vi "FPGA_main_simplified_debug.vi"() -> ()   [LabVIEW 2024]
uses:
  <vilib>/Platform/TimedLoop/XDataNode/timing_clust.ctl
  <vilib>/Platform/TimedLoop/XDataNode/nitl_modes.ctl
  <vilib>/Platform/TimedLoop/XDataNode/wakeup.ctl
  <vilib>/LabVIEW Targets/FPGA/cRIO/shared/nicrio_ModuleControls/nicrio_cRIO-9775_ContinuousDataRates4ChansRing.ctl
  <vilib>/rvi/Emulation/niFpgaGetClockAttributes.vi
  <vilib>/rvi/Emulation/niFpgaSctlEmulationGetInTimedLoop.vi
  <vilib>/rvi/Emulation/niFpgaEmulationReportErrorSimple.vi
  <vilib>/rvi/Emulation/niFpgaProcessEmulError.vi
  <vilib>/rvi/eio/common/nirviEmuTemplateMethod_errors.vi
  <vilib>/rvi/Emulation/niFpgaCriticalErrorInLSC.vi
  <vilib>/rvi/eio/common/nirviEmuTemplatePropertySet_errors.vi
  <vilib>/eio/utilities/niEioResolveVilibRelativePath.vi
  <vilib>/rvi/interface/RandomDataEmulation/niFpgaRandomDataHandleErrors.vi
  <vilib>/eio/EIONode/EIONode.xnode
  <vilib>/eio/EIOMethodNode/EIOMethodNode.xnode
  <vilib>/eio/EIOPropertyNode/EIOPropertyNode.xnode
  <vilib>/platform/TimedLoop/XDataNode/XDataNode.xnode
  <vilib>/rvi/DataTransferAndStorage/Container/XNode/niFpgaContainer.xnode
  <vilib>/rvi/interface/RandomDataEmulation/nirviRandomDataFpgaReadWriteTemplate.vi
  <vilib>/Platform/TimedLoop/XDataNode/XDNodeRunTimeDep.lvlib
  <vilib>/rvi/eio/common/nirviEmuTemplatePropertyGet_errors.vi
  <vilib>/rvi/eio/common/nirviEmuTemplatePropertyGet_noerrors.vi
  <vilib>/rvi/eio/common/nirviEmuTemplatePropertySet_noerrors.vi
panel:
  out "Use Triggers":bool
  out "Tr FIFO Full":bool
  out "@Next R":u32
  out "Last Tr (R-F)":u32
  out "Current Data Cycle":u32
  out "Tr Finished":bool
  in  "Total Triggers":u32=10
  out "Current Trigger":u32
  out "FPGA routine\nrunning":bool
  in  "Pulse\nWidth":u32 caption="Pulse width(uSec)"
  in  "Pulse\nPeriod":u32 caption="Period(uSec)"
  in  "Stop Routine":bool
  in  "DIO3":bool
  in  "DIO2":bool
  in  "DIO1":bool
  in  "DIO0":bool
  out "Rebinned Counts":i32
  in  "Binning Time (ticks)":i32=1200000
  out "Counts":u8
  out "FPGA Error":errorcluster
  out "Finished":bool
  in  "Stop":bool
  out "Module Underflow":bool
  out "DMA FIFO Full":bool
  out "Actual Loop Period (ticks)":u32=40
  out "First Read":bool
  in  "Type Counter":enum16{"Falling Edge", "Rising Edge"}(ring)
  # "Photon counting. Single cycle time loop"
  # "User Control of digital output"
  # "Thresholding"
  # "Pulsing DIO 0 (Pulse width should be shorter than\n period)"
  # "Binning and streaming binned Total Count"
  # "Streaming Analog Input Data"
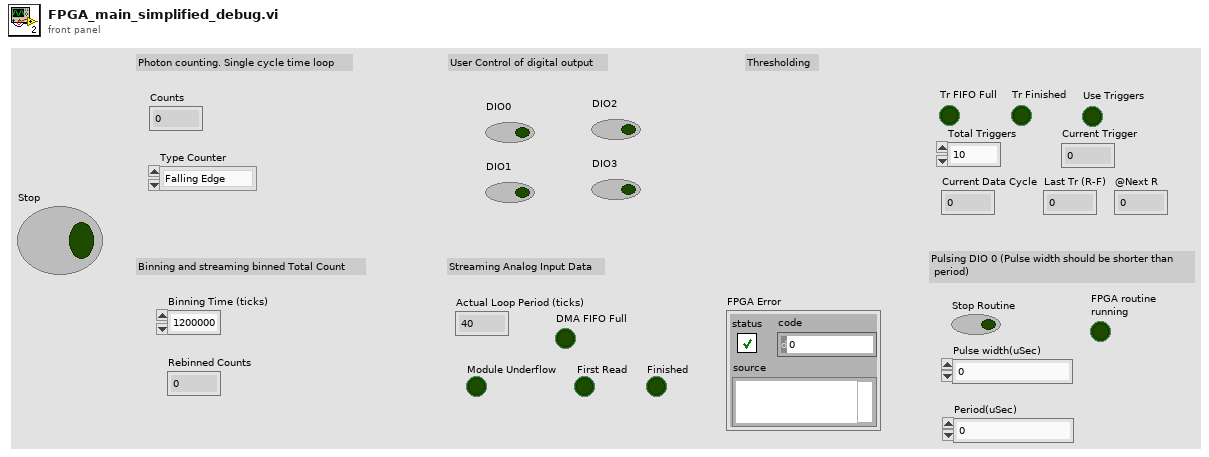
[diagram p1: front panel]
types:
  T1 = typedef "XDNodeRunTimeDep.lvlib/timing_clust.ctl" = cluster{"Expected End [f-1]":u64, "Actual End [f-1]":u64, "Finished Late? [f-1]":bool, "Expected End [i-1]":u64, "Actual End [i-1]":u64, "Finished Late? [i-1]":bool, "Expected Start [i]":u64, "Actual Start [i]":u64, "Expected Start [f]":u64, "Actual Start [f]":u64, "Source Name":string, "Structure Name":string, "Period":i64, "Deadline":i64, "Offset":i64, "Start":i64, "Priority":i32, "Timeout":i32, "Mode":T2, "Wakeup Reason":T3, "Error":errorcluster, "Source Type":string, "Secondary Source Type":string, "Global End Time":u64, "Global Start Time":u64, "Frame Duration":u64, "Iteration Duration":u64, "Assigned CPU":i32, "I/O Scan Engine Mode":u32}
  T2 = typedef "XDNodeRunTimeDep.lvlib/nitl_modes.ctl" = enum32{"No Change", "Process missed periods, maintain original phase", "Discard missed periods, maintain original phase", "Process missed periods, ignore original phase", "Discard missed periods, ignore original phase"}
  T3 = typedef "XDNodeRunTimeDep.lvlib/wakeup.ctl" = enum32{"Normal", "Aborted", "Asynchronous wakeup", "Timing source error", "Timed loop error", "Timeout"}
  T4 = typedef "nicrio_cRIO-9775_ContinuousDataRates4ChansRing.ctl" = u16
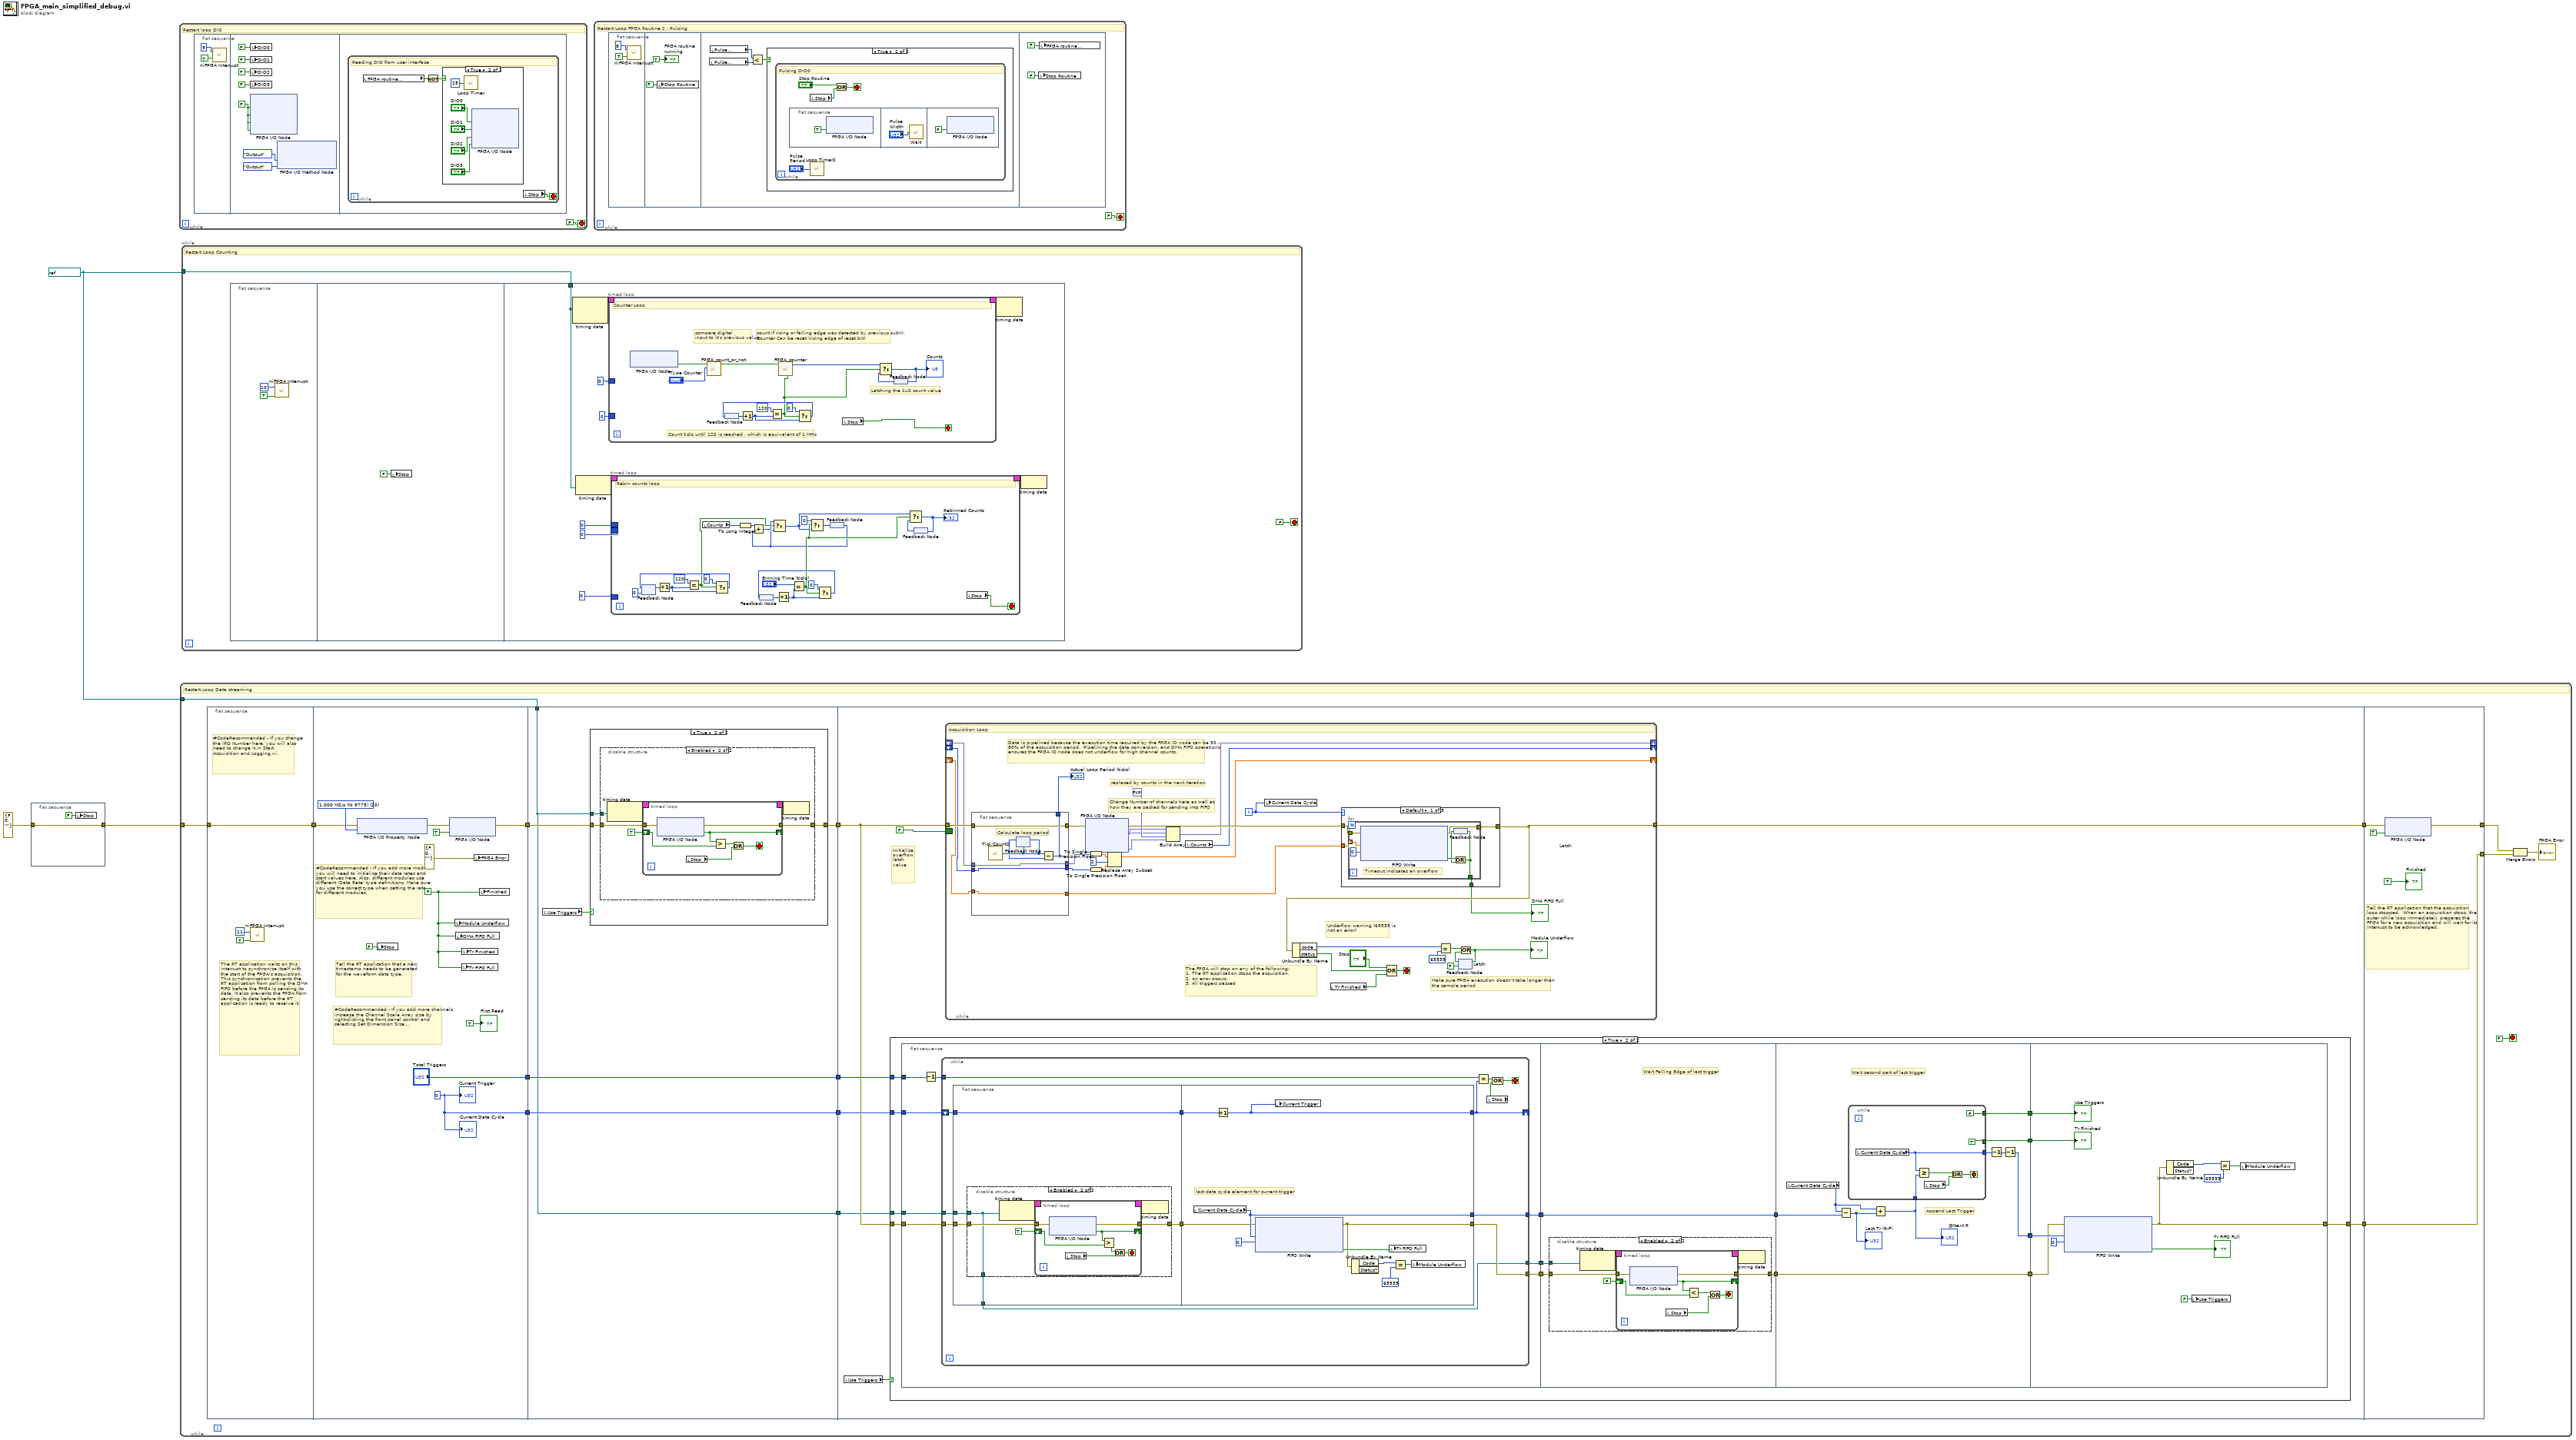
[diagram p0: block diagram]
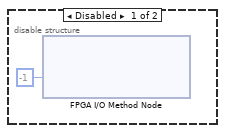
[diagram p3: hidden frame]
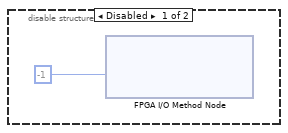
[diagram p5: hidden frame]
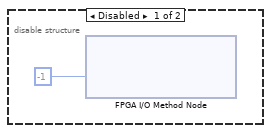
[diagram p6: hidden frame]
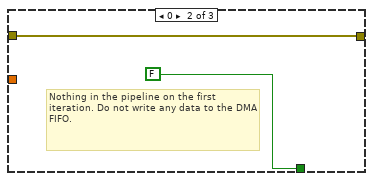
[diagram p7: hidden frame]
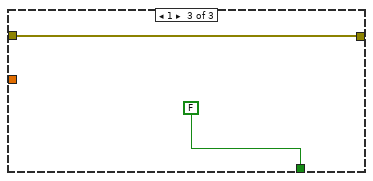
[diagram p8: hidden frame]
diagram:
  w1 = refnum<k21> "120MHz" ("Source Name")
  n1 = flat-sequence {
    tunnel: errorcluster {"status"=FALSE, "code"=0, "source"=""} ("Error") -> [w4]
    tunnel: [w4] -> w2
    frame #0 {
      n2 = local write "Stop"(FALSE ("stop")) -> ()
    }
  }
  n3 = while {
    stop <- FALSE stop-if-true
    # "Restart loop DIO"
    n4 = flat-sequence {
      frame #0 {
        n5 = call <vilib>:"niFPGA Interrupt.vi"("Wait Until Cleared (F)"=TRUE ("Wait Until Cleared"), "IRQ Number (0)"=u8 9 ("IRQ Number")) -> ()  [unwired: 1 in]
      }
      frame #1 {
        w11 = FALSE ("Mod3/DIO0")
        n6 = local write "DIO0"(FALSE ("DIO0")) -> ()
        n7 = local write "DIO1"(FALSE ("DIO1")) -> ()
        n8 = local write "DIO2"(FALSE ("DIO2")) -> ()
        n9 = local write "DIO3"(FALSE ("DIO3")) -> ()
        n10 = xnode "FPGA I/O Node"("Mod3/DIO0"=w11, "Mod3/DIO1"=w11, "Mod3/DIO2"=w11, "Mod3/DIO3"=w11) -> ()  [unwired: 4 in, 4 out]
        n11 = xnode "FPGA I/O Method Node"("DIO 7:4"=enum8{"No Change", "Input", "Output"}."Output", "DIO 3:0"=enum8{"No Change", "Input", "Output"}."Output") -> ()  [unwired: 1 in, 1 out]
      }
      frame #2 {
        n12 = while {
          stop <- w18 stop-if-true
          # "Reading DIO from user interface"
          n13 = local read "FPGA routine\nrunning"() -> (w17:bool)
          n14 = Not(x=w17) -> (.not. x?=w16:bool)
          n15 = case shown="True" w16 {
            frame False {
            }
            frame True {
              n16 = call "Loop Timer"("Count(mSec)"=u8 25) -> ()  [unwired: 1 out]
              n17 = xnode "FPGA I/O Node"("Mod3/DIO0"="DIO0", "Mod3/DIO1"="DIO1", "Mod3/DIO2"="DIO2", "Mod3/DIO3"="DIO3") -> ()  [unwired: 4 in, 4 out]
            }
          }
          n18 = local read "Stop"() -> (w18:bool)
        }
      }
    }
  }
  n19 = while {
    tunnel: w2 -> [w37]
    tunnel: w1 -> [w26]
    stop <- FALSE stop-if-true
    # "Restart Loop Data streaming"
    n20 = flat-sequence {
      tunnel: w37 -> [w40]
      tunnel: [w40] -> w27
      tunnel: [w44] -> w34
      tunnel: ["Total Triggers"] -> w32
      tunnel: [w48] -> w31
      tunnel: w27 -> [w46]
      tunnel: [w56] -> w36
      tunnel: [w59] -> w35
      tunnel: w34 -> [w59]
      tunnel: [w58] -> w33
      tunnel: w32 -> [w58]
      tunnel: w31 -> [w57]
      tunnel: w26 -> [w55]
      tunnel: [w55] -> w25
      tunnel: w36 -> [w87]
      tunnel: [w90] -> w38
      tunnel: w35 -> [w89]
      tunnel: w33 -> [w88]
      tunnel: [w86] -> w30
      tunnel: w25 -> [w85]
      tunnel: w38 -> [w273]
      tunnel: [w272] -> w29
      tunnel: w30 -> [w271]
      tunnel: [w271] -> w28
      frame #0 {
        # "#CodeRecommended - If you change the IRQ Number here, you will also need to change it in Start Acquisition and Logging.vi."
        # "The RT application waits on this interrupt to synchronize itself with the start of the FPGA's acquisition.  This synchronization prevents the RT application from polling the DMA FIFO before the FPGA is sending its data. It also prevents the FPGA from sending its data before the RT application is ready to receive it."
        n21 = call <vilib>:"niFPGA Interrupt.vi"("Wait Until Cleared (F)"=TRUE ("Wait Until Cleared"), "IRQ Number (0)"=u8 11 ("IRQ Number")) -> ()  [unwired: 1 in]
      }
      frame #1 {
        w44 = u32 0 ("Current Trigger")
        w50 = T4 20 items=["1.000 MS/s (NI 9775)"=20, "833.333 KS/s (NI 9775)"=24, "714.286 KS/s (NI 9775)"=28, "625.000 KS/s (NI 9775)"=32, "555.556 KS/s (NI 9775)"=36, "500.000 KS/s (NI 9775)"=40, "454.545 KS/s (NI 9775)"=44, "416.667 KS/s (NI 9775)"=48, "384.615 KS/s (NI 9775)"=52, "357.143 KS/s (NI 9775)"=56, "333.333 KS/s (NI 9775)"=60, "312.500 KS/s (NI 9775)"=64, "294.118 KS/s (NI 9775)"=68, "277.778 KS/s (NI 9775)"=72, "263.158 KS/s (NI 9775)"=76, "250.000 KS/s (NI 9775)"=80, "238.095 KS/s (NI 9775)"=84, "227.273 KS/s (NI 9775)"=88, "217.391 KS/s (NI 9775)"=92, "208.333 KS/s (NI 9775)"=96, "200.000 KS/s (NI 9775)"=100, "192.308 KS/s (NI 9775)"=104, "185.185 KS/s (NI 9775)"=108, "178.571 KS/s (NI 9775)"=112, "172.414 KS/s (NI 9775)"=116, "166.667 KS/s (NI 9775)"=120, "161.290 KS/s (NI 9775)"=124, "156.250 KS/s (NI 9775)"=128, "151.515 KS/s (NI 9775)"=132, "147.059 KS/s (NI 9775)"=136, "142.857 KS/s (NI 9775)"=140, "138.889 KS/s (NI 9775)"=144, "135.135 KS/s (NI 9775)"=148, "131.579 KS/s (NI 9775)"=152, "128.205 KS/s (NI 9775)"=156, "125.000 KS/s (NI 9775)"=160, "121.951 KS/s (NI 9775)"=164, "119.048 KS/s (NI 9775)"=168, "116.279 KS/s (NI 9775)"=172, "113.636 KS/s (NI 9775)"=176, "111.111 KS/s (NI 9775)"=180, "108.696 KS/s (NI 9775)"=184, "106.383 KS/s (NI 9775)"=188, "104.167 KS/s (NI 9775)"=192, "102.041 KS/s (NI 9775)"=196, "100.000 KS/s (NI 9775)"=200, "50.000 KS/s (NI 9775)"=400, "33.333 KS/s (NI 9775)"=600, "25.000 KS/s (NI 9775)"=800, "20.000 KS/s (NI 9775)"=1000, "16.667 KS/s (NI 9775)"=1200, "14.286 KS/s (NI 9775)"=1400, "12.500 KS/s (NI 9775)"=1600, "11.111 KS/s (NI 9775)"=1800, "10.000 KS/s (NI 9775)"=2000, "9.091 KS/s (NI 9775)"=2200, "8.333 KS/s (NI 9775)"=2400, "7.692 KS/s (NI 9775)"=2600, "7.143 KS/s (NI 9775)"=2800, "6.667 KS/s (NI 9775)"=3000, "6.250 KS/s (NI 9775)"=3200, "5.882 KS/s (NI 9775)"=3400, "5.556 KS/s (NI 9775)"=3600, "5.000 KS/s (NI 9775)"=4000, "4.762 KS/s (NI 9775)"=4200, "4.545 KS/s (NI 9775)"=4400, "4.348 KS/s (NI 9775)"=4600, "4.167 KS/s (NI 9775)"=4800, "4.000 KS/s (NI 9775)"=5000, "3.846 KS/s (NI 9775)"=5200, "3.571 KS/s (NI 9775)"=5600, "3.333 KS/s (NI 9775)"=6000, "3.125 KS/s (NI 9775)"=6400, "2.941 KS/s (NI 9775)"=6800, "2.778 KS/s (NI 9775)"=7200, "2.632 KS/s (NI 9775)"=7600, "2.500 KS/s (NI 9775)"=8000, "2.381 KS/s (NI 9775)"=8400, "2.273 KS/s (NI 9775)"=8800, "2.174 KS/s (NI 9775)"=9200, "2.083 KS/s (NI 9775)"=9600, "2.000 KS/s (NI 9775)"=10000, "1.923 KS/s (NI 9775)"=10400, "1.852 KS/s (NI 9775)"=10800, "1.786 KS/s (NI 9775)"=11200, "1.724 KS/s (NI 9775)"=11600, "1.667 KS/s (NI 9775)"=12000, "1.613 KS/s (NI 9775)"=12400, "1.563 KS/s (NI 9775)"=12800, "1.515 KS/s (NI 9775)"=13200, "1.471 KS/s (NI 9775)"=13600, "1.429 KS/s (NI 9775)"=14000, "1.389 KS/s (NI 9775)"=14400, "1.351 KS/s (NI 9775)"=14800, "1.316 KS/s (NI 9775)"=15200, "1.282 KS/s (NI 9775)"=15600, "1.250 KS/s (NI 9775)"=16000, "1.220 KS/s (NI 9775)"=16400, "1.190 KS/s (NI 9775)"=16800, "1.163 KS/s (NI 9775)"=17200, "1.136 KS/s (NI 9775)"=17600, "1.111 KS/s (NI 9775)"=18000, "1.087 KS/s (NI 9775)"=18400, "1.064 KS/s (NI 9775)"=18800, "1.042 KS/s (NI 9775)"=19200, "1.020 KS/s (NI 9775)"=19600, "1.000 KS/s (NI 9775)"=20000, "0.980 KS/s (NI 9775)"=20400, "0.962 KS/s (NI 9775)"=20800, "0.943 KS/s (NI 9775)"=21200, "0.926 KS/s (NI 9775)"=21600, "0.909 KS/s (NI 9775)"=22000, "0.893 KS/s (NI 9775)"=22400, "0.877 KS/s (NI 9775)"=22800, "0.862 KS/s (NI 9775)"=23200, "0.847 KS/s (NI 9775)"=23600, "0.833 KS/s (NI 9775)"=24000, "0.820 KS/s (NI 9775)"=24400, "0.806 KS/s (NI 9775)"=24800, "0.794 KS/s (NI 9775)"=25200, "0.781 KS/s (NI 9775)"=25600, "0.694 KS/s (NI 9775)"=28800, "0.625 KS/s (NI 9775)"=32000, "0.568 KS/s (NI 9775)"=35200, "0.521 KS/s (NI 9775)"=38400, "0.446 KS/s (NI 9775)"=44800, "0.391 KS/s (NI 9775)"=51200, "0.347 KS/s (NI 9775)"=57600, "0.313 KS/s (NI 9775)"=64000] ("Continuous Data Rate")
        w47 = FALSE ("Module Underflow")
        # "Tell the RT application that a new timestamp needs to be generated for the waveform data type."
        # "#CodeRecommended - If you add more channels, increase the Channel Scale Array size by right-clicking the front panel control and selecting Set Dimension Size..."
        # "#CodeRecommended - If you add more modules, you will need to initialize their data rates and start values here. Also, different modules use different 'Data Rate' type definitions. Make sure you use the correct type when setting the rate for different modules."
        n22 = xnode "FPGA I/O Property Node"("error in"=w46, "Continuous Data Rate"=w50) -> ("error out"=w51:errorcluster)  [unwired: 1 in, 1 out]
        n23 = local write "Stop"(FALSE ("Stop")) -> ()
        n24 = xnode "FPGA I/O Node"("error in"=w51, "Mod1/Start"=TRUE) -> ("error out"=w48:errorcluster)  [unwired: 1 in, 1 out]
        n25 = local write "Module Underflow"(w47) -> ()
        n26 = local write "DMA FIFO Full"(w47) -> ()
        n27 = local write "Tr FIFO Full"(w47) -> ()
        n28 = local write "Tr Finished"(w47) -> ()
        n29 = local write "FPGA Error"(errorcluster {"status"=FALSE, "code"=0, "source"=""} ("FPGA Error")) -> ()
        n30 = local write "Finished"(w47) -> ()
        "Current Trigger" <- w44
        "Current Data Cycle" <- w44
        "First Read" <- TRUE ("First Read")
      }
      frame #2 {
        n31 = local read "Use Triggers"() -> (w54:bool)
        n32 = case shown="True" w54 {
          tunnel: w57 -> [w60 w63]
          tunnel: [w60 w62] -> w56
          tunnel: w55 -> [_ w61]
          frame False {
          }
          frame True {
            n33 = disable-structure shown="Enabled" {
              disable-tunnel: w63 -> [_ w67]
              disable-tunnel: [_ w66] -> w62
              disable-tunnel: w61 -> [_ w65]
              frame Disabled {
                n34 = xnode "FPGA I/O Method Node"("Timeout"=-1) -> ()  [unwired: 1 in, 2 out]
              }
              frame Enabled {
                n35 = node-c288(w65) -> (w70:T1)
                n36 = timed-loop {
                  timing: w70 -> [_]
                  timing-out: [_] -> w69
                  shift-right: [w76] -> _
                  shift-left: TRUE ("Mod2/DIO2") -> [w77]
                  tunnel: w67 -> [w72]
                  tunnel: [w71] -> w66
                  stop <- w75 stop-if-true
                  n37 = xnode "FPGA I/O Node"("error in"=w72) -> ("error out"=w71:errorcluster, "Mod2/DIO2"=w76:bool)  [unwired: 1 in, 1 out]
                  n38 = local read "Stop"() -> (w73:bool)
                  n39 = Greater?(x=w76, y=w77) -> (0:w74:bool)
                  n40 = Or(x=w74, y=w73) -> (x .or. y?=w75:bool)
                }
                n41 = node-c288(w69) -> ()
              }
            }
          }
        }
      }
      frame #3 {
        # "Initialize overflow latch value"
        n42 = local read "Use Triggers"() -> (w84:bool)
        n43 = case shown="True" w84 {
          tunnel: w89 -> [_ w101]
          tunnel: w88 -> [_ w100]
          tunnel: w87 -> [w92 w99]
          tunnel: [w92 w98] -> w86
          tunnel: w85 -> [_ w97]
          frame False {
          }
          frame True {
            n44 = flat-sequence {
              tunnel: w101 -> [w114]
              tunnel: w100 -> [w112]
              tunnel: [w111] -> w106
              tunnel: w99 -> [w110]
              tunnel: [w109] -> w105
              tunnel: w97 -> [w108]
              tunnel: [w107] -> w104
              tunnel: w106 -> [w166]
              tunnel: [w166] -> w102
              tunnel: w105 -> [w165]
              tunnel: [w164] -> w103
              tunnel: w104 -> [w163]
              tunnel: w103 -> [w189]
              tunnel: w102 -> [w193]
              tunnel: [w190] -> w96
              tunnel: [w189] -> w95
              tunnel: [w188] -> w94
              tunnel: [w187] -> w93
              tunnel: [w206] -> w98
              tunnel: w96 -> [w209]
              tunnel: w95 -> [w207]
              tunnel: w94 -> [w205]
              tunnel: w93 -> [w204]
              frame #0 {
                n45 = Decrement(x=w112) -> (x-1=w113:u32)
                n46 = while {
                  shift-right: [w125] -> _
                  shift-left: w114 -> [w127]
                  tunnel: w113 -> [w124]
                  tunnel: [w123] -> w111
                  tunnel: w110 -> [w119]
                  tunnel: [w118] -> w109
                  tunnel: w108 -> [w116]
                  tunnel: [w115] -> w107
                  stop <- w122 stop-if-true
                  n47 = flat-sequence {
                    tunnel: w127 -> [w132]
                    tunnel: [w132] -> w126
                    tunnel: w119 -> [w131]
                    tunnel: [w130] -> w117
                    tunnel: w116 -> [w129]
                    tunnel: [w128] -> w115
                    tunnel: [w162] -> w125
                    tunnel: w126 -> [w161]
                    tunnel: [w159] -> w123
                    tunnel: [w154] -> w118
                    tunnel: w117 -> [w158]
                    frame #0 {
                      n48 = disable-structure shown="Enabled" {
                        disable-tunnel: w131 -> [_ w136]
                        disable-tunnel: [_ w135] -> w130
                        disable-tunnel: w129 -> [_ w134]
                        disable-tunnel: [_ w134] -> w128
                        frame Disabled {
                          n49 = xnode "FPGA I/O Method Node"("Timeout"=-1) -> ()  [unwired: 1 in, 2 out]
                        }
                        frame Enabled {
                          n50 = node-c288(w134) -> (w139:T1)
                          n51 = timed-loop {
                            timing: w139 -> [_]
                            timing-out: [_] -> w138
                            shift-right: [w145] -> _
                            shift-left: TRUE ("Mod2/DIO2") -> [w146]
                            tunnel: w136 -> [w141]
                            tunnel: [w140] -> w135
                            stop <- w144 stop-if-true
                            n52 = xnode "FPGA I/O Node"("error in"=w141) -> ("error out"=w140:errorcluster, "Mod2/DIO2"=w145:bool)  [unwired: 1 in, 1 out]
                            n53 = local read "Stop"() -> (w142:bool)
                            n54 = Greater?(x=w145, y=w146) -> (0:w143:bool)
                            n55 = Or(x=w143, y=w142) -> (x .or. y?=w144:bool)
                          }
                          n56 = node-c288(w138) -> ()
                        }
                      }
                    }
                    frame #1 {
                      # "last data cycle element for current trigger"
                      n57 = local read "Current Data Cycle"() -> (w159:u32)
                      n58 = Increment(x=w161) -> (x+1=w162:u32)
                      n59 = xnode ("FIFO Write")("Element"=w159, "Timeout"=0, "error in (no error)"=w158) -> ("Timed Out?"=w157:bool, "error out"=w154:errorcluster)  [unwired: 1 in, 1 out]
                      n60 = local write "Current Trigger"(w162) -> ()
                      n61 = Unbundle By Name(w154) -> ("Code"=w155:i32)  [unwired: 1 out]
                      n62 = local write "Tr FIFO Full"(w157) -> ()
                      n63 = Equal?(x=w155, y=65539) -> (x = y?=w153:bool)
                      n64 = local write "Module Underflow"(w153) -> ()
                    }
                  }
                  n65 = Equal?(x=w124, y=w125) -> (x = y?=w121:bool)
                  n66 = local read "Stop"() -> (w120:bool)
                  n67 = Compound Arithmetic op=OR(w121, w120) -> (w122:bool)
                }
              }
              frame #1 {
                # "Wait Falling Edge of last trigger"
                n68 = disable-structure shown="Enabled" {
                  disable-tunnel: w165 -> [_ w170]
                  disable-tunnel: [_ w169] -> w164
                  disable-tunnel: w163 -> [_ w168]
                  frame Disabled {
                    n69 = xnode "FPGA I/O Method Node"("Timeout"=-1) -> ()  [unwired: 1 in, 2 out]
                  }
                  frame Enabled {
                    n70 = node-c288(w168) -> (w173:T1)
                    n71 = timed-loop {
                      timing: w173 -> [_]
                      timing-out: [_] -> w172
                      shift-right: [w178] -> _
                      shift-left: FALSE ("Mod2/DIO2") -> [w179]
                      tunnel: w170 -> [w175]
                      tunnel: [w174] -> w169
                      stop <- w177 stop-if-true
                      n72 = xnode "FPGA I/O Node"("error in"=w175) -> ("error out"=w174:errorcluster, "Mod2/DIO2"=w178:bool)  [unwired: 1 in, 1 out]
                      n73 = local read "Stop"() -> (w176:bool)
                      n74 = Less?(x=w178, y=w179) -> (x < y?=w180:bool)
                      n75 = Or(x=w180, y=w176) -> (x .or. y?=w177:bool)
                    }
                    n76 = node-c288(w172) -> ()
                  }
                }
              }
              frame #2 {
                # "Wait second part of last trigger"
                # "Append Last Trigger"
                n77 = local read "Current Data Cycle"() -> (w195:u32)
                n78 = Subtract(x=w195, y=w193) -> (x-y=w196:u32)
                "Last Tr (R-F)" <- w196
                n79 = Add(x=w195, y=w196) -> (x+y=w194:u32)
                "@Next R" <- w194
                n80 = while {
                  tunnel: w194 -> [w203]
                  tunnel: [w202] -> w192
                  tunnel: [TRUE] -> w188
                  tunnel: [FALSE] -> w187
                  stop <- w200 stop-if-true
                  n81 = local read "Current Data Cycle"() -> (w202:u32)
                  n82 = Greater Or Equal?(x=w202, y=w203) -> (x >= y?=w199:bool)
                  n83 = local read "Stop"() -> (w198:bool)
                  n84 = Or(x=w199, y=w198) -> (x .or. y?=w200:bool)
                }
                n85 = Decrement(x=w192) -> (x-1=w191:u32)
                n86 = Decrement(x=w191) -> (x-1=w190:u32)
              }
              frame #3 {
                n87 = xnode ("FIFO Write")("Element"=w209, "Timeout"=0, "error in (no error)"=w207) -> ("Timed Out?"=→"Tr FIFO Full":bool, "error out"=w206:errorcluster)  [unwired: 1 in, 1 out]
                n88 = Unbundle By Name(w206) -> ("Code"=w212:i32)  [unwired: 1 out]
                n89 = local write "Use Triggers"(FALSE ("Use Triggers")) -> ()
                n90 = Equal?(x=w212, y=65539) -> (x = y?=w213:bool)
                n91 = local write "Module Underflow"(w213) -> ()
                "Tr Finished" <- w205
                "Use Triggers" <- w204
              }
            }
          }
        }
        n92 = while {
          tunnel: w87 -> [w243]
          tunnel: [w247] -> w90
          border: FALSE ("Overflow\nLatch") -> [_]
          shift-right: [w235] -> _
          shift-left: _ -> [w234]
          shift-right: [w226] -> _
          shift-left: _ -> [w232]
          shift-right: [w223] -> _
          shift-left: _ -> [w231]
          i -> [w221]
          stop <- w246 stop-if-true
          # "replaced by counts in the next iteration"
          # "Data is pipelined because the execution time required by the FPGA IO node can be 50 - 80% of the acquisition period.  Pipelining the data conversion, and DMA FIFO operations ensures the FPGA IO node does not underflow for high channel counts."
          # "Change Number of channels here as well as \nhow they are packed for sending into FIFO"
          # "Underflow warning (65539 is not an error)"
          # "The FPGA will stop on any of the following:\n1. The RT application stops the acquisition.\n2. An error occurs.\n3. All triggers passed"
          # "Make sure FPGA execution doesn't take longer than the sample period"
          # "Acquisition Loop"
          n93 = flat-sequence {
            tunnel: [w269] -> w242
            tunnel: w243 -> [w269]
            tunnel: [w266] -> w216
            tunnel: w234 -> [w265]
            tunnel: [w265] -> w233
            tunnel: w232 -> [w264]
            tunnel: [w264] -> w220
            tunnel: w231 -> [w263]
            tunnel: [w263] -> w230
            frame #0 {
              # "Calculate loop period"
              n94 = call "Tick Count2"() -> ("Tick Count(Ticks)"=w268:u32)
              n95 = feedback-in #1(w268) -> ()
              n96 = feedback #1(w268) -> (w267:u32)
              n97 = Subtract(x=w268, y=w267) -> (x-y=w266:u32)
            }
          }
          n98 = xnode "FPGA I/O Node"("error in"=w242) -> ("error out"=w236:errorcluster, "Mod1/AI0"=w225:fxp<+/-,17,5>, "Mod1/AI1"=w224:fxp<+/-,17,5>, "Mod1/AI2"=w215:fxp<+/-,17,5>)  [unwired: 3 in, 3 out]
          n99 = To Single Precision Float(number=w233) -> (single precision float=w229:sgl[])
          n100 = To Single Precision Float(number=w230) -> (single precision float=w227:sgl)
          n101 = Replace Array Subset(array=w229, new element=w227, index=2) -> (w226:sgl[])
          n102 = Build Array(w225, w224, fxp<+/-,17,5> 0.0 ("element"), w215) -> (w235:fxp<+/-,17,5>[])
          n103 = local read "Counts"() -> (w223:u8)
          n104 = local write "Current Data Cycle"(w221) -> ()
          n105 = local read "Tr Finished"() -> (w222:bool)
          n106 = case shown="Default" w221 {
            tunnel: [w248 FALSE FALSE] -> w218
            tunnel: w220 -> [w251 _ _]
            tunnel: w236 -> [w250 w259 w261]
            tunnel: [w249 w259 w261] -> w247
            frame Default {
              n107 = for {
                tunnel: [w256] -> w248
                tunnel: w251 -> [w252] mode=indexing
                tunnel: w250 -> [w254]
                tunnel: [w253] -> w249
                # "Timeout indicates an overflow"
                n108 = xnode ("FIFO Write")("Element"=w252, "Timeout"=0, "error in (no error)"=w254) -> ("Timed Out?"=w258:bool, "error out"=w253:errorcluster)  [unwired: 1 in, 1 out]
                n109 = feedback #2 "Latch"() -> (w257:bool)
                n110 = Or(x=w258, y=w257) -> (x .or. y?=w256:bool)
                n111 = feedback-in #2(w256) -> ()
              }
            }
            frame 0 {
              # "Nothing in the pipeline on the first iteration. Do not write any data to the DMA FIFO."
            }
            frame 1 {
            }
          }
          "DMA FIFO Full" <- w218
          n112 = Unbundle By Name(w247) -> ("code"=w244:i32, "status"=w238:bool)
          n113 = Compound Arithmetic op=OR("Stop", w238, w222) -> (w246:bool)
          n114 = Equal?(x=w244, y=65539) -> (x = y?=w239:bool)
          n115 = feedback #3 "Latch"(FALSE) -> (w241:bool)
          n116 = Or(x=w239, y=w241) -> (x .or. y?=w217:bool)
          "Module Underflow" <- w217
          n117 = feedback-in #3(w217) -> ()
          "Actual Loop Period (ticks)" <- w216
        }
      }
      frame #4 {
        # "Tell the RT application that the acquisition loop stopped.  When an acquisition stops, the outer while loop immediately prepares the FPGA for a new acquisition and will wait for its interrupt to be acknowledged."
        n118 = xnode "FPGA I/O Node"("error in"=w273, "Mod1/Stop"=TRUE) -> ("error out"=w272:errorcluster)  [unwired: 1 in, 1 out]
        "Finished" <- TRUE ("Finished")
      }
    }
    n119 = Merge Errors(w29, w28) -> (→"FPGA Error":errorcluster)
  }
  n120 = while {
    tunnel: w1 -> [w275]
    stop <- FALSE stop-if-true
    # "Restart Loop Counting"
    n121 = flat-sequence {
      tunnel: w275 -> [w280]
      frame #0 {
        n122 = call <vilib>:"niFPGA Interrupt.vi"("Wait Until Cleared (F)"=TRUE ("Wait Until Cleared"), "IRQ Number (0)"=u8 10 ("IRQ Number")) -> ()  [unwired: 1 in]
      }
      frame #1 {
        n123 = local write "Stop"(FALSE ("Stop")) -> ()
      }
      frame #2 {
        n124 = node-c288(w280) -> (w289:T1)  [unwired: 1 in]
        n125 = node-c288(w280) -> (w285:T1)
        n126 = timed-loop {
          timing: w289 -> [_]
          timing-out: [_] -> w288
          border: u8 0 ("t") -> [_]
          border: u8 0 ("Total Count") -> [_]
          stop <- w319 stop-if-true
          # "Latching the 1uS count value"
          # "Count ticks until 120 is reached , which is equivalent of 1 MHz"
          # "count if rising or falling edge was detected by previous subVI. Counter Can be reset (rising edge of reset bit)"
          # "compare digital\ninput to it's previous value"
          # "Counter Loop"
          n127 = xnode "FPGA I/O Node"() -> ("Mod2/DIO0"=w330:bool)  [unwired: 1 in, 1 out]
          n128 = call "FPGA_count_or_not.vi"("Type Counter"="Type Counter", "Countable"=w330) -> ("Count or Not?"=w331:bool)  [unwired: 9 in]
          n129 = feedback #4() -> (w328:u8)
          n130 = Increment(x=w328) -> (x+1=w326:u8)
          n131 = Equal?(x=u8 120 ("y"), y=w326) -> (x = y?=w323:bool)
          n132 = call "FPGA_counter.vi"("Count or Not?"=w331, "Reset Photon Count"=w323) -> ("Total Count"=w322:u8)  [unwired: 8 in]
          n133 = Select(t=u8 0, s=w323, f=w326) -> (s? t:f=w324:u8)
          n134 = feedback-in #4(w324) -> ()
          n135 = local read "Stop"() -> (w319:bool)
          n136 = feedback #5() -> (w320:u8)
          n137 = Select(t=w322, s=w323, f=w320) -> (s? t:f=w321:u8)
          "Counts" <- w321
          n138 = feedback-in #5(w321) -> ()
        }
        n139 = timed-loop {
          timing: w285 -> [_]
          timing-out: [_] -> w284
          border: 0 ("Counts") -> [_]
          border: 0 ("t") -> [_]
          border: 0 -> [_]
          stop <- w302 stop-if-true
          # "Rebin counts loop"
          n140 = feedback #6(u8 0 ("t")) -> (w299:u8)
          n141 = Increment(x=w299) -> (x+1=w297:u8)
          n142 = Equal?(x=u8 120 ("y"), y=w297) -> (x = y?=w292:bool)
          n143 = local read "Counts"() -> (w301:u8)
          n144 = Select(t=u8 0, s=w292, f=w297) -> (s? t:f=w295:u8)
          n145 = feedback-in #6(w295) -> ()
          n146 = To Long Integer(number=w301) -> (32bit integer=w300:i32)
          n147 = feedback #7() -> (w309:i32)
          n148 = Increment(x=w309) -> (x+1=w310:i32)
          n149 = Equal?(x="Binning Time (ticks)", y=w310) -> (x = y?=w305:bool)
          n150 = Select(t=0, s=w305, f=w310) -> (s? t:f=w312:i32)
          n151 = feedback-in #7(w312) -> ()
          n152 = feedback #8() -> (w293:i32)
          n153 = Add(x=w300, y=w293) -> (x+y=w294:i32)
          n154 = Select(t=w294, s=w292, f=w293) -> (s? t:f=w290:i32)
          n155 = Select(t=0, s=w305, f=w290) -> (s? t:f=w304:i32)
          n156 = feedback-in #8(w304) -> ()
          n157 = feedback #9() -> (w306:i32)
          n158 = Select(t=w290, s=w305, f=w306) -> (s? t:f=w307:i32)
          "Rebinned Counts" <- w307
          n159 = feedback-in #9(w307) -> ()
          n160 = local read "Stop"() -> (w302:bool)
        }
        n161 = node-c288(w288) -> ()  [unwired: 1 out]
        n162 = node-c288(w284) -> ()
      }
    }
  }
  n163 = while {
    stop <- FALSE stop-if-true
    # "Restart Loop FPGA Routine 1 : Pulsing"
    n164 = flat-sequence {
      frame #0 {
        n165 = call <vilib>:"niFPGA Interrupt.vi"("Wait Until Cleared (F)"=TRUE ("Wait Until Cleared"), "IRQ Number (0)"=u8 8 ("IRQ Number")) -> ()  [unwired: 1 in]
      }
      frame #1 {
        n166 = local write "Stop Routine"(FALSE ("Stop Routine")) -> ()
        "FPGA routine\nrunning" <- TRUE
      }
      frame #2 {
        n167 = local read "Pulse\nPeriod"() -> (w344:u32)
        n168 = local read "Pulse\nWidth"() -> (w345:u32)
        n169 = Less?(x=w345, y=w344) -> (x < y?=w343:bool)
        n170 = case shown="True" w343 {
          frame False {
          }
          frame True {
            n171 = while {
              stop <- w348 stop-if-true
              # "Pulsing DIO0"
              n172 = flat-sequence {
                frame #0 {
                  n173 = xnode "FPGA I/O Node"("Mod3/DIO0"=TRUE) -> ()  [unwired: 1 in, 1 out]
                }
                frame #1 {
                  n174 = call "Wait"("Count(uSec)"="Pulse\nWidth") -> ()  [unwired: 1 out]
                }
                frame #2 {
                  n175 = xnode "FPGA I/O Node"("Mod3/DIO0"=FALSE) -> ()  [unwired: 1 in, 1 out]
                }
              }
              n176 = local read "Stop"() -> (w349:bool)
              n177 = call "Loop Timer2"("Count(uSec)"="Pulse\nPeriod") -> ()  [unwired: 1 out]
              n178 = Or(x="Stop Routine", y=w349) -> (x .or. y?=w348:bool)
            }
          }
        }
      }
      frame #3 {
        n179 = local write "Stop Routine"(FALSE ("Stop Routine")) -> ()
        n180 = local write "FPGA routine\nrunning"(FALSE ("FPGA routine\nrunning")) -> ()
      }
    }
  }
